vi "Steam.vi"() -> ()   [LabVIEW 2013]
panel:
  out "Steam Interlock":bool
  out "TI-322":dbl
  out "Boolean 4":bool
  in  "Steam":bool
  in  "FT-310":dbl
  out "TI-321":dbl format="%.1f"
  out "TI-331":dbl format="%.1f"
  out "PI-321":dbl format="%.1f"
  out "TI-341":dbl format="%.1f"
  out "TI-342":dbl
  # "HX-340"
  # "HX-330"
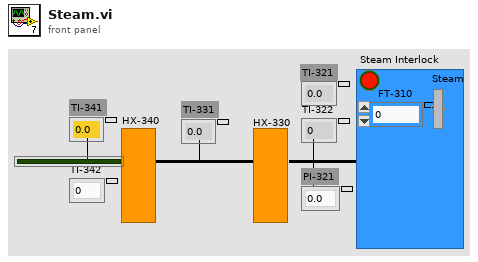
[diagram p1: front panel]
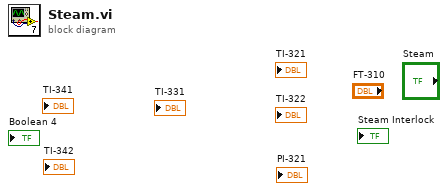
[diagram p0: block diagram]
diagram:
